vi "EXTI_IO_ISR.vi"(11 "Interrupt_Flag":T1) -> ()   [LabVIEW 2011]
uses:
  D:/National Instruments/LabVIEW 2011/Targets/Keil/Embedded/RealView/Generic/My_ARM_Starter_Board/STM32_DriverVI_Interface/Interrupt/Interrupt_ISR.ctl
  <vilib>/eio/EIO_TerminalDirection.ctl
  <vilib>/STM32_DriverVI_Interface_F4/Interrupt/Interrupt_Flag_F4.ctl
  <vilib>/STM32_DriverVI_Interface_F4/GPIO_EIO/GPI_EIO_Inner_F4.vi
  <vilib>/STM32_DriverVI_Interface_F4/GPIO_EIO/GPO_EIO_Inner_F4.vi
  <vilib>/eio/EIONode/EIONode.xnode
panel:
  # "说明：\n这是一个标准的中断模板 VI，用户可以直接使用,\n在相应的Case语句里面实现相应的中断服务程序即可！\n\n双击打开这个VI之后，另存为副本，名称不变，将其保存\n并添加到自己的项目浏览器中，然后在程序生成规范中进行\n属性设置！"
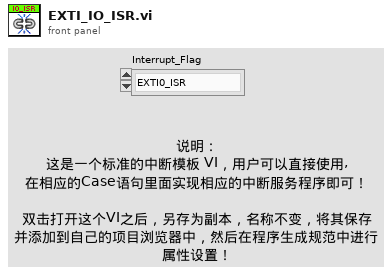
[diagram p1: front panel]
types:
  T1 = typedef "Interrupt_ISR.ctl" = enum8{"EXTI0_ISR", "EXTI1_ISR", "EXTI2_ISR", "EXTI3_ISR", "EXTI4_ISR", "EXTI5_ISR", "EXTI6_ISR", "EXTI7_ISR", "EXTI8_ISR", "EXTI9_ISR", "EXTI10_ISR", "EXTI11_ISR", "EXTI12_ISR", "EXTI13_ISR", "EXTI14_ISR", "EXTI15_ISR"}
  T2 = enum8{"P0", "P1", "P2", "P3", "P4", "P5", "P6", "P7", "P8", "P9", "P10", "P11", "P12", "P13", "P14", "P15"}
  T3 = typedef "Interrupt_Flag_F4.ctl" = enum8{"EXTI0_Flag", "EXTI1_Flag", "EXTI2_Flag", "EXTI3_Flag", "EXTI4_Flag", "EXTI5_Flag", "EXTI6_Flag", "EXTI7_Flag", "EXTI8_Flag", "EXTI9_Flag", "EXTI10_Flag", "EXTI11_Flag", "EXTI12_Flag", "EXTI13_Flag", "EXTI14_Flag", "EXTI15_Flag"}
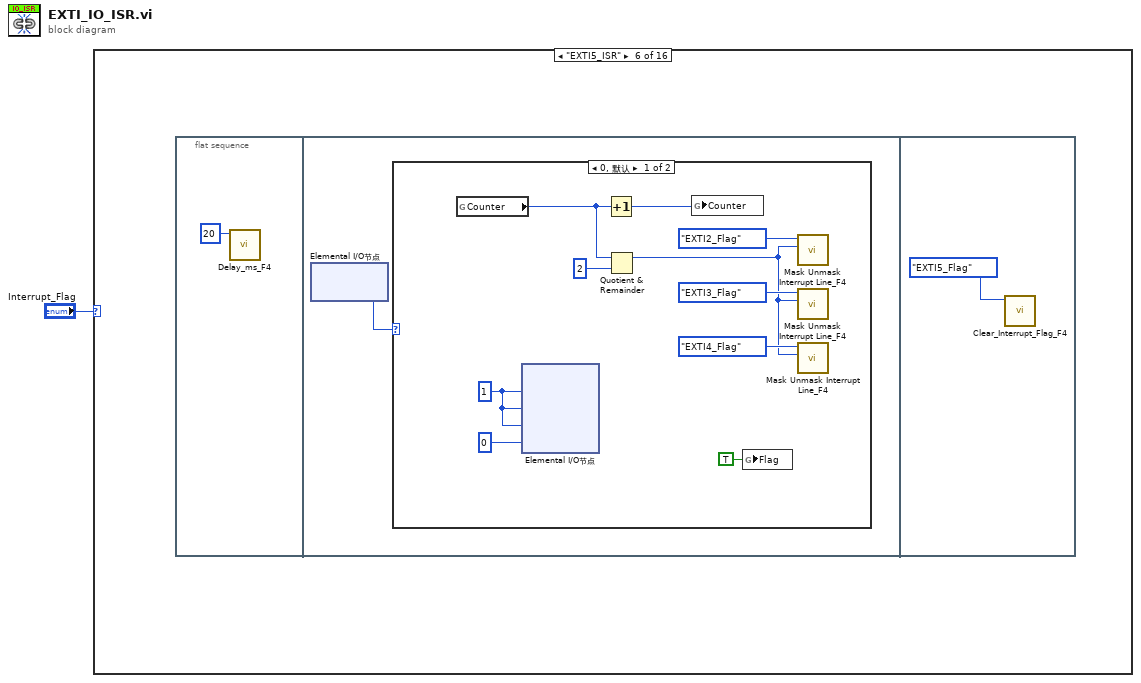
[diagram p0: block diagram]
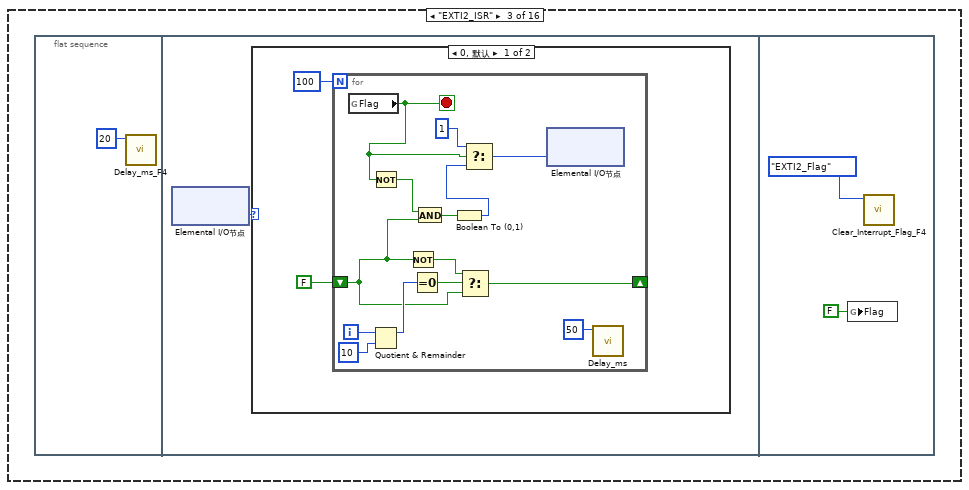
[diagram p4: hidden frame]
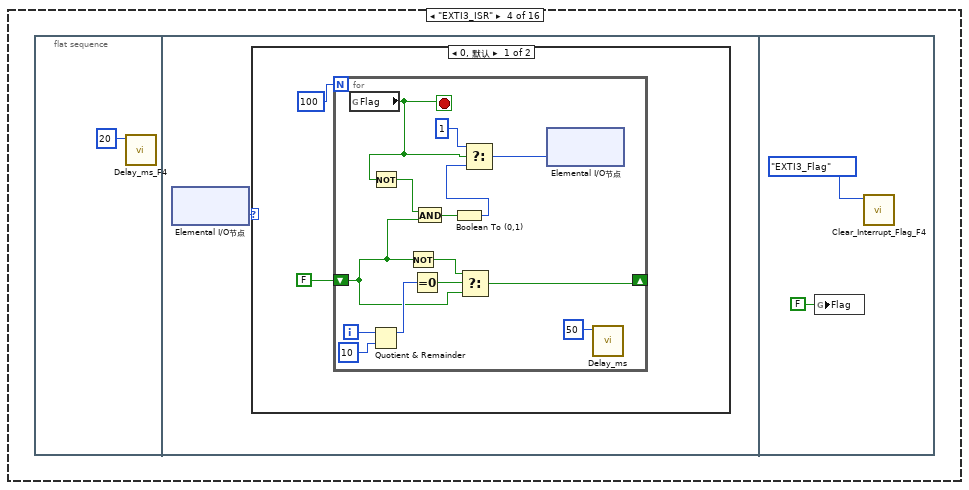
[diagram p6: hidden frame]
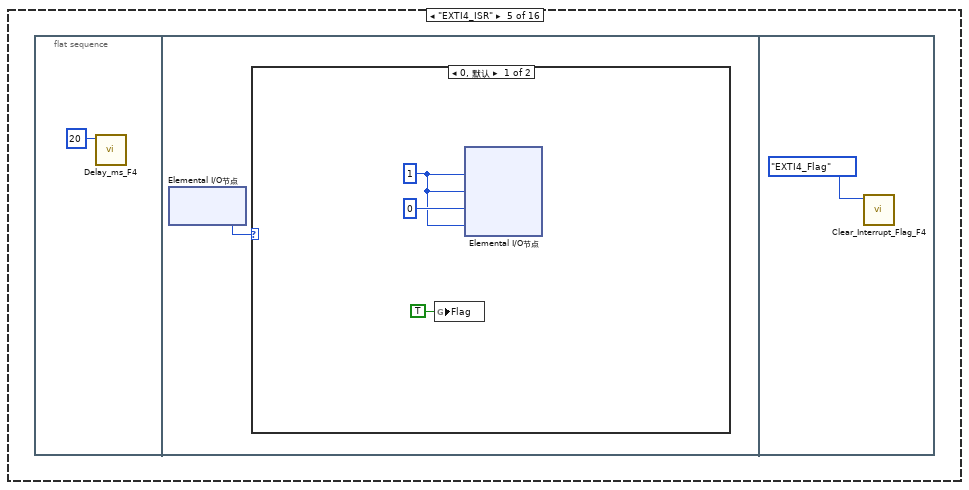
[diagram p8: hidden frame]
diagram:
  n1 = case shown="\"EXTI5_ISR\"" "Interrupt_Flag" {
    frame "EXTI0_ISR", Default {
      n2 = flat-sequence {
        frame #0 {
          # "添加自己的中断服务程序"
        }
        frame #1 {
          # "别忘了添加\n清除中断标志：ISR完成了"
        }
      }
    }
    frame "EXTI1_ISR" {
    }
    frame "EXTI2_ISR" {
      n3 = flat-sequence {
        frame #0 {
          n4 = call <vilib>:"Delay_ms_F4.vi"("time_ms"=u32 20) -> ()  [unwired: 10 in, 1 out]
        }
        frame #1 {
          n5 = xnode "Elemental I/O节点"() -> ("KEY_1"=w3:u8)  [unwired: 1 in, 1 out]
          n6 = case shown="0, 默认" w3 {
            frame 0, Default {
              n7 = for {
                N: 100 -> [_]
                shift-right: [w11] -> _
                shift-left: FALSE -> [w17]
                i -> [w22]
                stop <- w10 stop-if-true
                n8 = global read "全局变量.vi" "Flag"() -> (w10:bool)
                n9 = Not(x=w10) -> (.not. x?=w14:bool)
                n10 = Quotient & Remainder(x=w22, y=10) -> (x-y*floor(x/y)=w20:i32)  [unwired: 1 out]
                n11 = Not(x=w17) -> (.not. x?=w18:bool)
                n12 = Equal To 0?(x=w20) -> (x = 0?=w19:bool)
                n13 = And(x=w14, y=w17) -> (x .and. y?=w16:bool)
                n14 = Boolean To (0,1)(Boolean=w16) -> (0, 1=w15:i16)
                n15 = Select(t=w18, s=w19, f=w17) -> (s? t:f=w11:bool)
                n16 = Select(t=i16 1, s=w10, f=w15) -> (s? t:f=w12:i16)
                n17 = xnode "Elemental I/O节点"("LED_1"=w12) -> ()  [unwired: 1 in, 1 out]
                n18 = call <vilib>:"Delay_ms.vi"("time_ms"=u16 50) -> ()  [unwired: 10 in, 1 out]
              }
            }
            frame 1 {
            }
          }
        }
        frame #2 {
          n19 = global write "全局变量.vi" "Flag"(FALSE ("Flag")) -> ()
          n20 = call <vilib>:"Clear_Interrupt_Flag_F4.vi"("中断标志位"=Interrupt_Flag_F4."EXTI2_Flag") -> ()  [unwired: 10 in, 1 out]
        }
      }
    }
    frame "EXTI3_ISR" {
      n21 = flat-sequence {
        frame #0 {
          n22 = call <vilib>:"Delay_ms_F4.vi"("time_ms"=u32 20) -> ()  [unwired: 10 in, 1 out]
        }
        frame #1 {
          n23 = xnode "Elemental I/O节点"() -> ("KEY_2"=w31:u8)  [unwired: 1 in, 1 out]
          n24 = case shown="0, 默认" w31 {
            frame 0, Default {
              n25 = for {
                N: 100 -> [_]
                shift-right: [w39] -> _
                shift-left: FALSE -> [w45]
                i -> [w50]
                stop <- w38 stop-if-true
                n26 = global read "全局变量.vi" "Flag"() -> (w38:bool)
                n27 = Not(x=w38) -> (.not. x?=w42:bool)
                n28 = Quotient & Remainder(x=w50, y=10) -> (x-y*floor(x/y)=w48:i32)  [unwired: 1 out]
                n29 = Not(x=w45) -> (.not. x?=w46:bool)
                n30 = Equal To 0?(x=w48) -> (x = 0?=w47:bool)
                n31 = And(x=w42, y=w45) -> (x .and. y?=w44:bool)
                n32 = Boolean To (0,1)(Boolean=w44) -> (0, 1=w43:i16)
                n33 = Select(t=w46, s=w47, f=w45) -> (s? t:f=w39:bool)
                n34 = Select(t=i16 1, s=w38, f=w43) -> (s? t:f=w40:i16)
                n35 = xnode "Elemental I/O节点"("LED_2"=w40) -> ()  [unwired: 1 in, 1 out]
                n36 = call <vilib>:"Delay_ms.vi"("time_ms"=u16 50) -> ()  [unwired: 10 in, 1 out]
              }
            }
            frame 1 {
            }
          }
        }
        frame #2 {
          n37 = global write "全局变量.vi" "Flag"(FALSE ("Flag")) -> ()
          n38 = call <vilib>:"Clear_Interrupt_Flag_F4.vi"("中断标志位"=Interrupt_Flag_F4."EXTI3_Flag") -> ()  [unwired: 10 in, 1 out]
        }
      }
    }
    frame "EXTI4_ISR" {
      n39 = flat-sequence {
        frame #0 {
          n40 = call <vilib>:"Delay_ms_F4.vi"("time_ms"=u32 20) -> ()  [unwired: 10 in, 1 out]
        }
        frame #1 {
          n41 = xnode "Elemental I/O节点"() -> ("KEY_3"=w59:u8)  [unwired: 1 in, 1 out]
          n42 = case shown="0, 默认" w59 {
            frame 0, Default {
              w65 = u8 1 ("LED_1")
              n43 = global write "全局变量.vi" "Flag"(TRUE ("Flag")) -> ()
              n44 = xnode "Elemental I/O节点"("LED_1"=w65, "LED_2"=w65, "LED_3"=u8 0 ("LED_4"), "LED_4"=w65) -> ()  [unwired: 4 in, 4 out]
            }
            frame 1 {
            }
          }
        }
        frame #2 {
          n45 = call <vilib>:"Clear_Interrupt_Flag_F4.vi"("中断标志位"=Interrupt_Flag_F4."EXTI4_Flag") -> ()  [unwired: 10 in, 1 out]
        }
      }
    }
    frame "EXTI5_ISR" {
      n46 = flat-sequence {
        frame #0 {
          n47 = call <vilib>:"Delay_ms_F4.vi"("time_ms"=u32 20) -> ()  [unwired: 10 in, 1 out]
        }
        frame #1 {
          n48 = xnode "Elemental I/O节点"() -> ("KEY_4"=w85:u8)  [unwired: 1 in, 1 out]
          n49 = case shown="0, 默认" w85 {
            frame 0, Default {
              w93 = u8 1 ("LED_1")
              n50 = global read "全局变量.vi" "Counter"() -> (w90:i32)
              n51 = xnode "Elemental I/O节点"("LED_1"=w93, "LED_2"=w93, "LED_3"=w93, "LED_4"=u8 0) -> ()  [unwired: 4 in, 4 out]
              n52 = Increment(x=w90) -> (x+1=w91:i32)
              n53 = Quotient & Remainder(x=w90, y=2) -> (x-y*floor(x/y)=w96:i32)  [unwired: 1 out]
              n54 = global write "全局变量.vi" "Counter"(w91) -> ()
              n55 = global write "全局变量.vi" "Flag"(TRUE ("Flag")) -> ()
              n56 = call <vilib>:"Mask Unmask Interrupt Line_F4.vi"("屏蔽或开启中断线"=w96, "IO中断线（标志位）"=Interrupt_Flag_F4."EXTI2_Flag") -> ()  [unwired: 9 in, 1 out]
              n57 = call <vilib>:"Mask Unmask Interrupt Line_F4.vi"("屏蔽或开启中断线"=w96, "IO中断线（标志位）"=Interrupt_Flag_F4."EXTI3_Flag") -> ()  [unwired: 9 in, 1 out]
              n58 = call <vilib>:"Mask Unmask Interrupt Line_F4.vi"("屏蔽或开启中断线"=w96, "IO中断线（标志位）"=Interrupt_Flag_F4."EXTI4_Flag") -> ()  [unwired: 9 in, 1 out]
            }
            frame 1 {
            }
          }
        }
        frame #2 {
          n59 = call <vilib>:"Clear_Interrupt_Flag_F4.vi"("中断标志位"=Interrupt_Flag_F4."EXTI5_Flag") -> ()  [unwired: 10 in, 1 out]
        }
      }
    }
    frame "EXTI6_ISR" {
    }
    frame "EXTI7_ISR" {
    }
    frame "EXTI8_ISR" {
    }
    frame "EXTI9_ISR" {
    }
    frame "EXTI10_ISR" {
    }
    frame "EXTI11_ISR" {
    }
    frame "EXTI12_ISR" {
    }
    frame "EXTI13_ISR" {
    }
    frame "EXTI14_ISR" {
    }
    frame "EXTI15_ISR" {
    }
  }
